vi "Constants.vi"() -> ()   [LabVIEW 2017]
panel:
  in  "ElevatorSetpoints":dbl[](array[numeric])=[11.0, 39.0, 90.0]
  in  "Track Width":dbl=29.0
  in  "CenterRotOffset":dbl=19.5
  in  "Height":dbl=38.5
  in  "Width":dbl=33.0
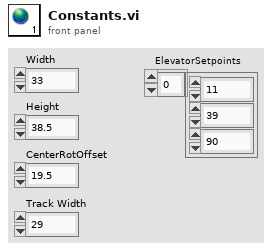
[diagram p1: front panel]
diagram:
